vi "TestGeneralSyntax.vi"(8 "error in (no error)":errorcluster) -> (0 "error out":errorcluster)   [LabVIEW 2019]
uses:
  <vilib>/addons/_JKI Toolkits/Caraya/classes/Test/Test.lvclass
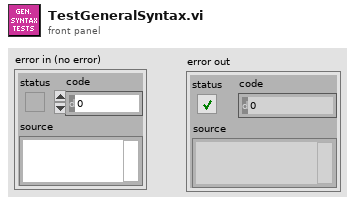
[diagram p1: front panel]
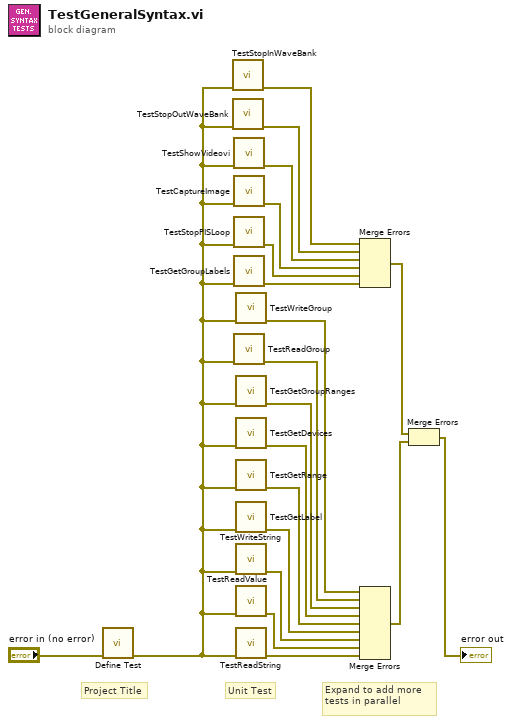
[diagram p0: block diagram]
diagram:
  # "Expand to add more tests in parallel"
  # "Unit Test"
  # "Project Title"
  n1 = call <vilib>:"Define Test.vi"("error in (no error)"="error in (no error)") -> ("error out"=w3:errorcluster)  [unwired: 10 in]
  n2 = call "TestStopInWaveBank.vi"("error in (no error)"=w3) -> ("error out"=w1:errorcluster)  [unwired: 10 in]
  n3 = call "TestStopOutWaveBank.vi"("error in (no error)"=w3) -> ("error out"=w2:errorcluster)  [unwired: 10 in]
  n4 = call "TestShowVideovi.vi"("error in (no error)"=w3) -> ("error out"=w4:errorcluster)  [unwired: 10 in]
  n5 = call "TestCaptureImage.vi"("error in (no error)"=w3) -> ("error out"=w5:errorcluster)  [unwired: 10 in]
  n6 = call "TestStopPISLoop.vi"("error in (no error)"=w3) -> ("error out"=w6:errorcluster)  [unwired: 10 in]
  n7 = call "TestGetGroupLabels.vi"("error in (no error)"=w3) -> ("error out"=w8:errorcluster)  [unwired: 10 in]
  n8 = call "TestReadGroup.vi"("error in (no error)"=w3) -> ("error out"=w12:errorcluster)  [unwired: 10 in]
  n9 = call "TestWriteGroup.vi"("error in (no error)"=w3) -> ("error out"=w11:errorcluster)  [unwired: 10 in]
  n10 = call "TestGetGroupRanges.vi"("error in (no error)"=w3) -> ("error out"=w13:errorcluster)  [unwired: 10 in]
  n11 = call "TestGetDevices.vi"("error in (no error)"=w3) -> ("error out"=w14:errorcluster)  [unwired: 10 in]
  n12 = call "TestGetRange.vi"("error in (no error)"=w3) -> ("error out"=w15:errorcluster)  [unwired: 10 in]
  n13 = call "TestGetLabel.vi"("error in (no error)"=w3) -> ("error out"=w16:errorcluster)  [unwired: 10 in]
  n14 = call "TestWriteString.vi"("error in (no error)"=w3) -> ("error out"=w17:errorcluster)  [unwired: 10 in]
  n15 = call "TestReadValue.vi"("error in (no error)"=w3) -> ("error out"=w18:errorcluster)  [unwired: 10 in]
  n16 = call "TestReadString.vi"("error in (no error)"=w3) -> ("error out"=w19:errorcluster)  [unwired: 10 in]
  n17 = Merge Errors(w1, w2, w4, w5, w6, w8) -> (w9:errorcluster)
  n18 = Merge Errors(w11, w12, w13, w14, w15, w16, w17, w18, w19) -> (w10:errorcluster)
  n19 = Merge Errors(w9, w10) -> (→"error out":errorcluster)
